vi "Generate Doc UID.vi"(8 "error in (no error)":errorcluster, 11 "Document in":refnum<class "Document.lvclass">) -> (0 "error out":errorcluster, 3 "Document out":refnum<class "Document.lvclass">)   [LabVIEW 2016, in "Document.lvclass"]
uses:
  Document.lvclass
  Document.lvclass/Document.ctl
  property/Write Doc UID.vi
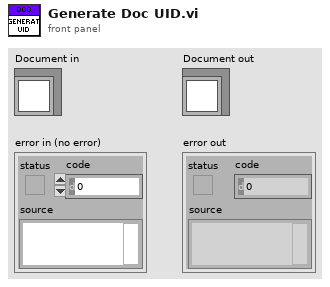
[diagram p1: front panel]
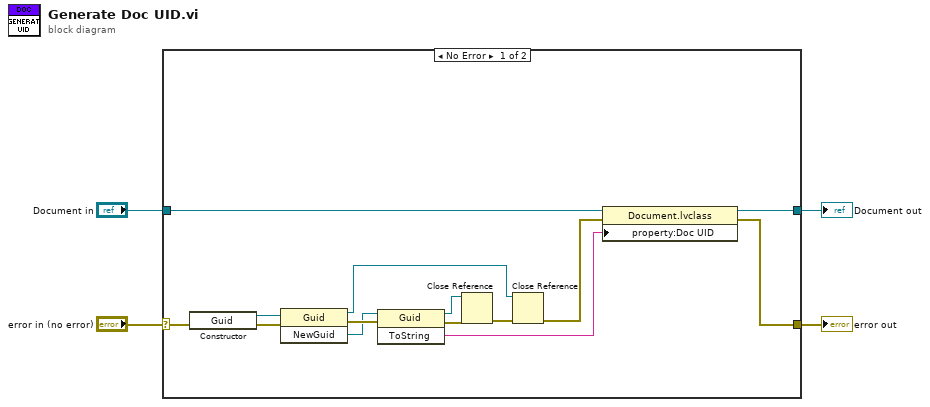
[diagram p0: block diagram]
diagram:
  n1 = case shown="No Error" "error in (no error)" {
    selector: "error in (no error)" -> [w11 w20]
    tunnel: [w10 w20] -> w3
    tunnel: [w12 w19] -> w1
    tunnel: "Document in" -> [w13 w19]
    frame No Error {
      n2 = constructor class="Guid"(error in=w11) -> (reference out=w15:refnum<k24>, error out=w16:errorcluster)  [unwired: 2 in, 1 out]
      n3 = invoke class="Guid" method="NewGuid"(reference=w15, error in=w16) -> (reference out=w6:refnum<k24>, error out=w18:errorcluster, "NewGuid"=w17:refnum<k24>)  [unwired: 1 in]
      n4 = invoke class="Guid" method="ToString"(reference=w17, error in=w18) -> (reference out=w8:refnum<k24>, error out=w9:errorcluster, "ToString"=w14:string)  [unwired: 1 in]
      n5 = Close Reference(reference=w8, error in (no error)=w9) -> (error out=w7:errorcluster)
      n6 = Close Reference(reference=w6, error in (no error)=w7) -> (error out=w5:errorcluster)
      n7 = property class="Document.lvclass"(reference=w13, error in=w5, "property:Doc UID"=w14) -> (reference out=w12:refnum<class "Document.lvclass">, error out=w10:errorcluster)
    }
    frame Error {
    }
  }
  "error out" <- w3
  "Document out" <- w1
